vi "tcp_服务器_发送.vi"(9 "远程端口或服务名称":u16=6314, 10 "原文件路径（使用对话框）":path=path "C:/Users/Administrator.2W964MZOGI5HE3B/Desktop/labview图片/105256rhad11pc5553vz5e.png", 11 "服务器网络地址":string="127.0.0.1") -> ()   [LabVIEW 2016, in "TCP文件传输系统.lvlib" / "TCP发送文件.lvlib"]
panel:
  out "当前步骤":T1(ring)
  out "error out":errorcluster
  out "错误输出":errorcluster
  out "已传百分比":string
  out "运行指示灯":bool
  in  "分帧数(兆)":i64=2
  out "侦数":i32
  out "已发帧数":i32
  out "在发第几次":i32
  out "共发送次数":string
  in  "分一包（兆）":i64=40
  out "文件名称":string
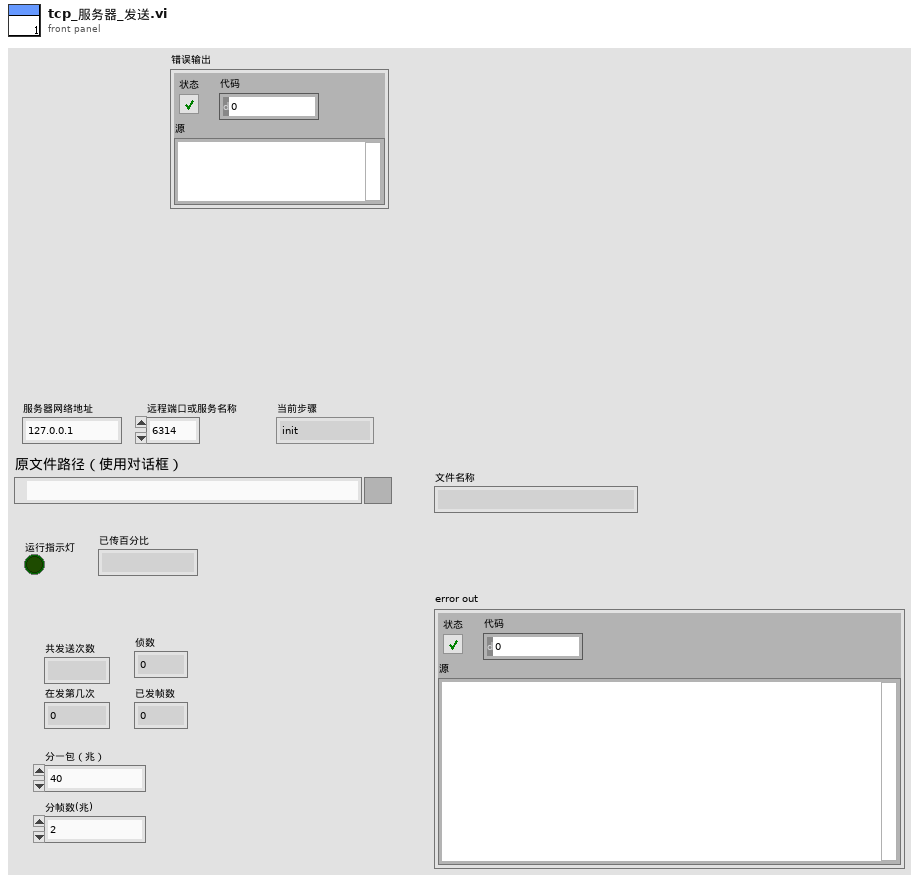
[diagram p1: front panel]
types:
  T1 = enum16{"init", "sendhead", "sendcontent", "sendsuccess", "over"}
  T2 = enum16{"open", "replace", "create", "open or create", "replace or create", "replace or create with confirmation"}
  T3 = cluster{"网络灯":bool, "发送中":bool, "已发送百分比":u8, "发送成功次数":dbl, "当前步骤":enum16{"init", "sendhead", "sendcontent", "sendsuccess", "over"}, "error out":errorcluster}
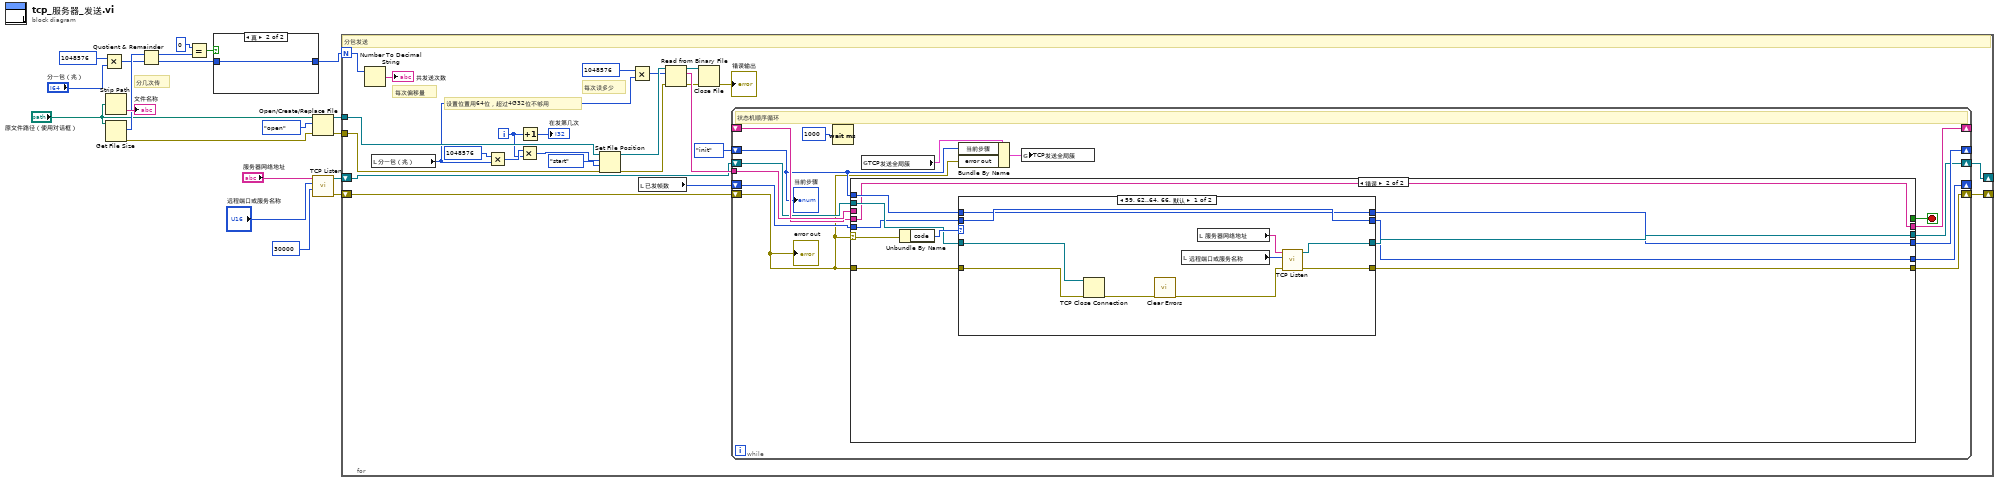
[diagram p0: block diagram]
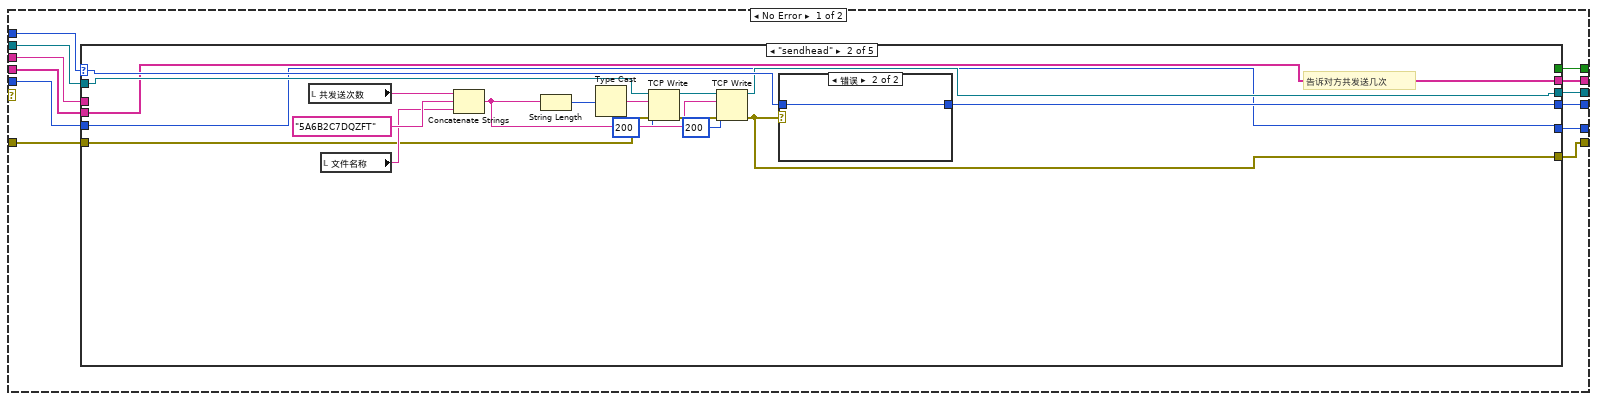
[diagram p2: hidden frame]
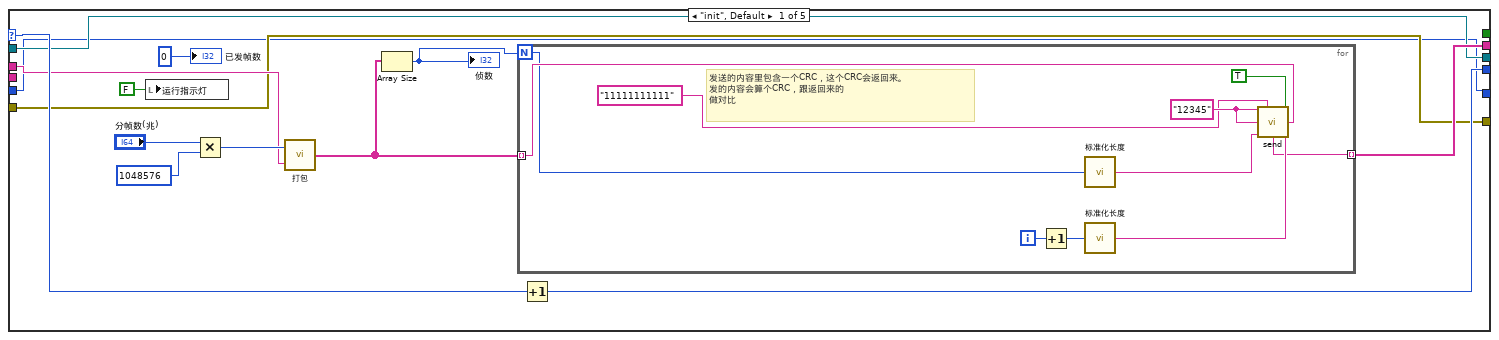
[diagram p3: hidden frame]
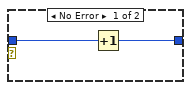
[diagram p4: hidden frame]
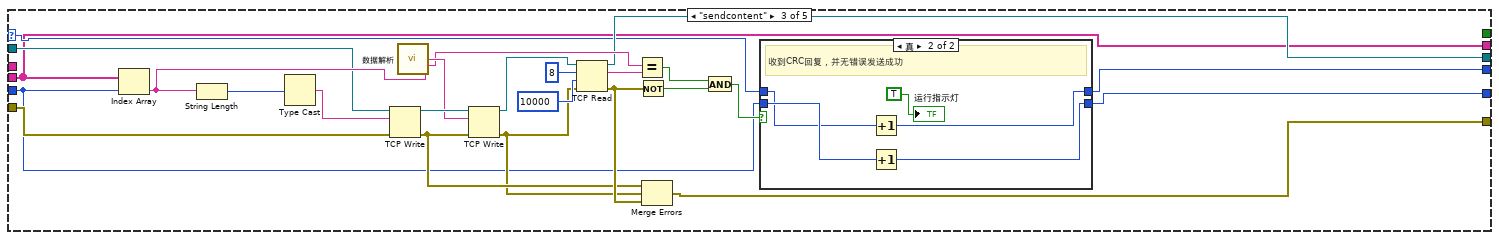
[diagram p5: hidden frame]
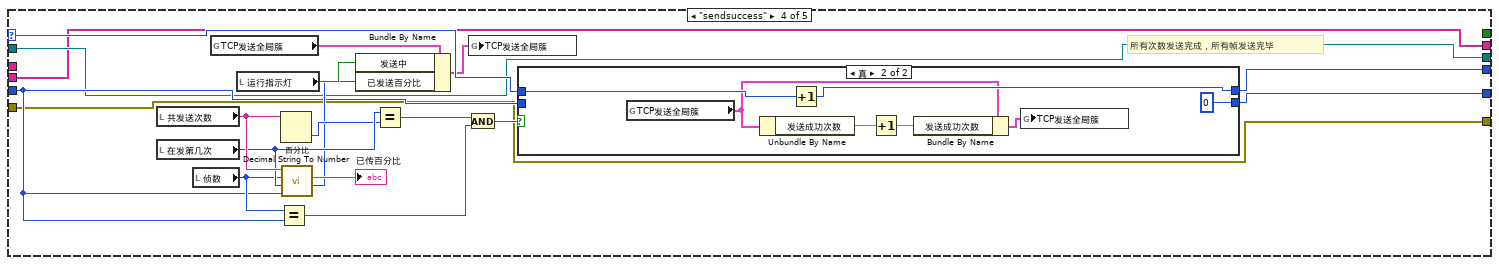
[diagram p7: hidden frame]
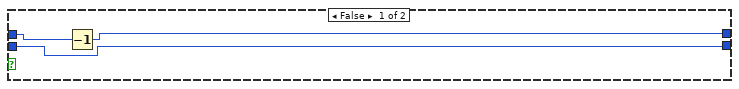
[diagram p8: hidden frame]
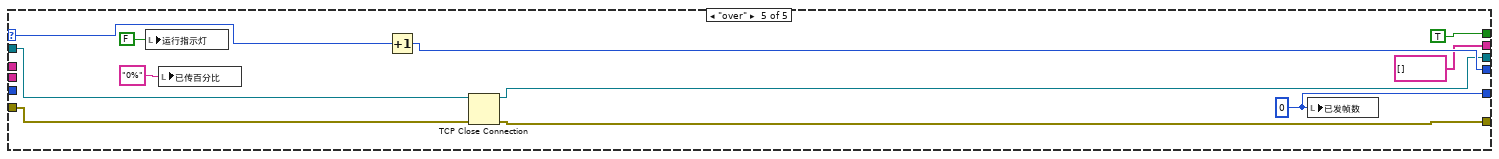
[diagram p9: hidden frame]
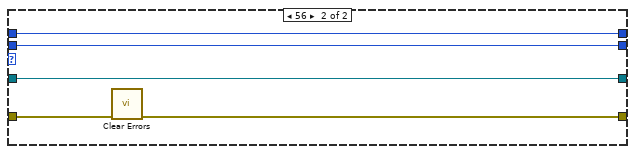
[diagram p10: hidden frame]
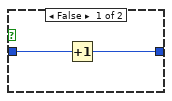
[diagram p11: hidden frame]
diagram:
  # "分几次传"
  n1 = Multiply(x=i64 1048576 ("y"), y="分一包（兆）") -> (x*y=w10:i64)
  n2 = Strip Path(path="原文件路径（使用对话框）") -> (name=→"文件名称":string)  [unwired: 1 out]
  n3 = Get File Size(file="原文件路径（使用对话框）") -> (size (in bytes)=w14:i64, 0:w15:errorcluster)  [unwired: 1 in, 1 out]
  n4 = Quotient & Remainder(x=w14, y=w10) -> (x-y*floor(x/y)=w19:i64, floor(x/y)=w16:i64)
  n5 = Equal?(x=0, y=w19) -> (x = y?=w17:bool)
  n6 = case shown="真" w17 {
    tunnel: [w21 w23] -> w8
    tunnel: w16 -> [w22 w23]
    frame False {
      n7 = Increment(x=w22) -> (x+1=w21:i64)
    }
    frame True {
    }
  }
  n8 = Open/Create/Replace File(file path (use dialog)="原文件路径（使用对话框）", error in=w15, operation (0:open)=T2."open" ("操作(0:open)")) -> (refnum out=w7:refnum<file>, error out=w6:errorcluster)  [unwired: 3 in, 1 out]
  n9 = call <vilib>:"TCP Listen.vi"("timeout ms (wait forever: -1)"=30000, "port"="远程端口或服务名称", "service name"="服务器网络地址") -> ("error out"=w3:errorcluster, "connection ID"=w4:refnum<k5>)  [unwired: 4 in, 3 out]
  n10 = for {
    N: w8 -> [w46]
    tunnel: w7 -> [w36]
    tunnel: w6 -> [w35]
    shift-right: [w29] -> _
    shift-left: w4 -> [w27]
    shift-right: [w28] -> _
    shift-left: w3 -> [w32]
    i -> [w34]
    # "设置位置用64位，超过4G32位不够用"
    # "每次读多少"
    # "每次偏移量"
    # "分包发送"
    n11 = Number To Decimal String(number=w46) -> (decimal integer string=→"共发送次数":string)  [unwired: 1 in]
    n12 = local read "分一包（兆）"() -> (w33:i64)
    n13 = Multiply(x=i64 1048576 ("偏移量（字节）（0）"), y=w33) -> (x*y=w39:i64)
    n14 = Multiply(x=w39, y=w34) -> (x*y=w42:i64)
    n15 = Increment(x=w34) -> (x+1=→"在发第几次":i32)
    n16 = Set File Position(offset (in bytes) (0)=w42, refnum=w36, from (0:start)=enum16{"start", "end", "current"}."start" ("自（0:起始）"), error in=w35) -> (refnum out=w44:refnum<file>, error out=w45:errorcluster)
    n17 = Multiply(x=1048576 ("总数(1)"), y=w33) -> (x*y=w37:i64)
    n18 = local read "已发帧数"() -> (w30:i32)
    n19 = Read from Binary File(8:w45, 10:w37, 11:w44) -> (0:w25:errorcluster, 2:w31:string, 3:w26:refnum<file>)  [unwired: 3 in, 1 out]
    n20 = Close File(refnum=w26, error in=w25) -> (error out=→"错误输出":errorcluster)  [unwired: 1 out]
    n21 = while {
      shift-right: [w63] -> _
      shift-left: T1."init" -> [w50]
      shift-right: [w58] -> w28
      shift-left: w32 -> [w49]
      tunnel: w31 -> [w60]
      shift-right: [w61] -> _
      shift-left: _ -> [w57]
      shift-right: [w55] -> _
      shift-left: w30 -> [w56]
      shift-right: [w59] -> w29
      shift-left: w27 -> [w54]
      stop <- w62 stop-if-true
      # "状态机顺序循环"
      n22 = Wait (ms)(milliseconds to wait=u32 1000 ("等待时间（毫秒）")) -> ()  [unwired: 1 out]
      n23 = case shown="错误" w49 {
        selector: w49 -> [_ w203]
        tunnel: w50 -> [w75 w197]
        tunnel: [w74 w196] -> w63
        tunnel: [w73 _] -> w62
        tunnel: [w72 w195] -> w61
        tunnel: w60 -> [w71 _]
        tunnel: w49 -> [w69 w201]
        tunnel: w54 -> [w70 w200]
        tunnel: [w66 w199] -> w59
        tunnel: [w67 w198] -> w58
        tunnel: w57 -> [w68 w195]
        tunnel: w56 -> [w65 w194]
        tunnel: [w64 w193] -> w55
        frame No Error {
          n24 = case shown="\"sendhead\"" w75 {
            selector: w75 -> [w89 w117 w123 w171 w192]
            tunnel: [w88 w116 w122 w170 w191] -> w74
            tunnel: [_ _ _ _ TRUE] -> w73
            tunnel: [w81 w105 w121 w153 string[] []] -> w72
            tunnel: w71 -> [w80 _ _ _ _]
            tunnel: w70 -> [w79 w107 w129 w155 w188]
            tunnel: w69 -> [w78 w106 w130 w154 w187]
            tunnel: w68 -> [_ w105 w121 w153 _]
            tunnel: [w78 w102 w127 w154 w185] -> w67
            tunnel: [w79 w104 w128 w155 w186] -> w66
            tunnel: w65 -> [w77 w103 w125 w156 _]
            tunnel: [w77 w103 w124 w157 w189] -> w64
            frame "init", Default {
              n25 = local write "运行指示灯"(FALSE ("运行指示灯")) -> ()
              n26 = Multiply(x="分帧数(兆)", y=i64 1048576) -> (x*y=w85:i64)
              n27 = call "打包.vi"("总内容"=w80, "分包大小"=w85) -> ("分包数组"=w84:string[])
              n28 = Array Size(array=w84) -> (size(s)=w86:i32)
              "侦数" <- w86
              n29 = for {
                N: w86 -> [w94]
                tunnel: w84 -> [w99] mode=indexing
                tunnel: [w92] -> w81 mode=indexing
                i -> [w98]
                w91 = "12345" ("内容说明（文件名）")
                # "发送的内容里包含一个CRC，这个CRC会返回来。\n发的内容会算个CRC，跟返回来的\n做对比"
                n30 = Increment(x=w98) -> (x+1=w93:i32)
                n31 = call "标准化长度.vi"("原长度"=w94) -> ("标准化长度"=w97:string)
                n32 = call "标准化长度.vi"("原长度"=w93) -> ("标准化长度"=w96:string)
                n33 = call "send.vi"("内容标识"=w91, "时标"="11111111111", "发送"=TRUE, "内容说明（文件名）"=w91, "帧内容"=w99, "帧数"=w97, "帧号"=w96) -> ("连接的字符串"=w92:string)  [unwired: 6 in, 2 out]
              }
              n34 = Increment(x=w89) -> (x+1=w88:T1)
              "已发帧数" <- 0 ("数值")
            }
            frame "sendhead" {
              # "告诉对方共发送几次"
              n35 = local read "共发送次数"() -> (w112:string)
              n36 = local read "文件名称"() -> (w113:string)
              n37 = Concatenate Strings(w112, "5A6B2C7DQZFT" ("字符串"), w113) -> (w108:string)
              n38 = String Length(string=w108) -> (length=w115:i32)
              n39 = Type Cast(x=w115) -> (*(type *) &x=w109:string)  [unwired: 1 out]
              n40 = TCP Write(connection ID=w107, data in=w109, error in (no error)=w106, 9:200 ("超时毫秒(25000)")) -> (connection ID out=w110:refnum<k5>, error out=w111:errorcluster)  [unwired: 1 out]
              n41 = TCP Write(connection ID=w110, data in=w108, error in (no error)=w111, 9:200 ("超时毫秒(25000)")) -> (connection ID out=w104:refnum<k5>, error out=w102:errorcluster)  [unwired: 1 out]
              n42 = case shown="错误" w102 {
                tunnel: w117 -> [w119 w120]
                tunnel: [w118 w120] -> w116
                frame No Error {
                  n43 = Increment(x=w119) -> (x+1=w118:T1)
                }
                frame Error {
                }
              }
            }
            frame "sendcontent" {
              n44 = Index Array(array=w121, index=w125) -> (element=w140:string)
              n45 = String Length(string=w140) -> (length=w144:i32)
              n46 = Type Cast(x=w144) -> (*(type *) &x=w141:string)  [unwired: 1 out]
              n47 = TCP Write(connection ID=w129, data in=w141, error in (no error)=w130) -> (connection ID out=w145:refnum<k5>, error out=w132:errorcluster)  [unwired: 2 out]
              n48 = call "数据解析.vi"("data in"=w140) -> ("data out"=w139:string, "CRC"=w137:string)  [unwired: 4 in, 9 out]
              n49 = TCP Write(connection ID=w145, data in=w139, error in (no error)=w132) -> (connection ID out=w143:refnum<k5>, error out=w131:errorcluster)  [unwired: 2 out]
              n50 = TCP Read(connection ID=w143, bytes to read=8 ("读取的字节"), error in (no error)=w131, 9:10000 ("超时毫秒(25000)")) -> (connection ID out=w128:refnum<k5>, data out=w138:string, error out=w133:errorcluster)  [unwired: 1 in]
              n51 = Equal?(x=w137, y=w138) -> (x = y?=w135:bool)
              n52 = Not(x=w133) -> (.not. x?=w134:bool)
              n53 = Merge Errors(w132, w131, w133) -> (w127:errorcluster)
              n54 = And(x=w135, y=w134) -> (x .and. y?=w126:bool)
              n55 = case shown="真" w126 {
                tunnel: w125 -> [w147 w151]
                tunnel: [w147 w150] -> w124
                tunnel: w123 -> [w146 w149]
                tunnel: [w146 w148] -> w122
                frame False {
                  # "未收到正确回复，或超时"
                }
                frame True {
                  # "收到CRC回复，并无错误发送成功"
                  n56 = Increment(x=w149) -> (x+1=w148:T1)
                  n57 = Increment(x=w151) -> (x+1=w150:i32)
                  "运行指示灯" <- TRUE
                }
              }
            }
            frame "sendsuccess" {
              # "所有次数发送完成，所有帧发送完毕"
              n58 = local read "共发送次数"() -> (w168:string)
              n59 = local read "在发第几次"() -> (w167:i32)
              n60 = local read "侦数"() -> (w165:i32)
              n61 = global read "全局变量1.vi" "TCP发送全局簇"() -> (w160:T3)
              n62 = local read "运行指示灯"() -> (w159:bool)
              n63 = Equal?(x=w165, y=w156) -> (x = y?=w163:bool)
              n64 = Decimal String To Number(string=w168) -> (number=w166:i32)  [unwired: 2 in, 1 out]
              n65 = call "百分比.vi"("已发帧数 2"=w156, "发第几次"=w167, "帧数"=w165, "共发送次数"=w168) -> ("已发送百分比"=w158:u8, "已传百分比"=→"已传百分比":string)  [unwired: 6 in]
              n66 = Bundle By Name(cluster=w160, "发送中"=w159, "已发送百分比"=w158) -> (w161:T3)
              n67 = Equal?(x=w167, y=w166) -> (x = y?=w164:bool)
              n68 = And(x=w164, y=w163) -> (x .and. y?=w162:bool)
              n69 = global write "全局变量1.vi" "TCP发送全局簇"(w161) -> ()
              n70 = case shown="真" w162 {
                tunnel: w171 -> [w174 w181]
                tunnel: [w173 w180] -> w170
                tunnel: [w172 0 ("已发帧数")] -> w157
                tunnel: w156 -> [w172 _]
                frame False {
                  n71 = Decrement(x=w174) -> (x-1=w173:T1)
                }
                frame True {
                  n72 = global read "全局变量1.vi" "TCP发送全局簇"() -> (w176:T3)
                  n73 = Unbundle By Name(w176) -> ("发送成功次数"=w177:dbl)
                  n74 = Increment(x=w181) -> (x+1=w180:T1)
                  n75 = Increment(x=w177) -> (x+1=w178:dbl)
                  n76 = Bundle By Name(cluster=w176, "发送成功次数"=w178) -> (w179:T3)
                  n77 = global write "全局变量1.vi" "TCP发送全局簇"(w179) -> ()
                }
              }
            }
            frame "over" {
              w189 = 0
              n78 = local write "运行指示灯"(FALSE ("运行指示灯")) -> ()
              n79 = local write "已传百分比"("0%" ("已传百分比")) -> ()
              n80 = Increment(x=w192) -> (x+1=w191:T1)
              n81 = TCP Close Connection(connection ID=w188, error in (no error)=w187) -> (connection ID out=w186:refnum<k5>, error out=w185:errorcluster)  [unwired: 1 in]
              n82 = local write "已发帧数"(w189) -> ()
            }
          }
        }
        frame Error {
          n83 = Unbundle By Name(w203) -> ("code"=w202:i32)
          n84 = case shown="59, 62..64, 66, 默认" w202 {
            tunnel: w201 -> [w213 w216]
            tunnel: w200 -> [w212 w215]
            tunnel: [w209 w215] -> w199
            tunnel: [w210 w214] -> w198
            tunnel: w197 -> [w208 w218]
            tunnel: [w208 w218] -> w196
            tunnel: w194 -> [w211 w217]
            tunnel: [w211 w217] -> w193
            frame 59, 62..64, 66, Default {
              n85 = TCP Close Connection(connection ID=w212, error in (no error)=w213) -> (error out=w207:errorcluster)  [unwired: 1 in, 1 out]
              n86 = call <vilib>:"Clear Errors.vi"("error in (no error)"=w207) -> ("error out"=w204:errorcluster)  [unwired: 5 in, 1 out]
              n87 = local read "远程端口或服务名称"() -> (w205:u16)
              n88 = local read "服务器网络地址"() -> (w206:string)
              n89 = call <vilib>:"TCP Listen.vi"("error in (no error)"=w204, "port"=w205, "service name"=w206) -> ("error out"=w210:errorcluster, "connection ID"=w209:refnum<k5>)  [unwired: 4 in, 3 out]
            }
            frame 56 {
              n90 = call <vilib>:"Clear Errors.vi"("error in (no error)"=w216) -> ("error out"=w214:errorcluster)  [unwired: 5 in, 1 out]
            }
          }
        }
      }
      n91 = global read "全局变量1.vi" "TCP发送全局簇"() -> (w52:T3)
      n92 = Bundle By Name(cluster=w52, "当前步骤"=w50, "error out"=w49) -> (w51:T3)
      n93 = global write "全局变量1.vi" "TCP发送全局簇"(w51) -> ()
      "error out" <- w49
      "当前步骤" <- w50
    }
  }
